vi "MATLAB - Cell Phone Towers.vi"() -> ()   [LabVIEW 2023]
doc: "This example illustrates the use of a Voronoi diagram by using radio towers. After 3 towers are placed, a Voronoi diagram is generated and overlayed to show the area of influence for each tower. It uses the 3D scene graph for display and covers such concepts as object creation, texturing, and transparency. A Voronoi diagram can also be used for path planning and obstacle avoidance in robotics."
panel:
  in  "voronoi output":T1
  out "3D Scene":refnum<vi>(3d-picture)
  in  "Tower height":sgl=3.0
  in  "Maximum amplitude":dbl=0.5
  in  "Size of terrain":i32=50
  in  "Stop":bool
  # "Overview: Illustrates the use of the MATLAB Node to compute a Voronoi diagram with cell phone towers.  After placing three towers, the Voronoi diagram appears.  Each location within a particular region should communicate with the cell phone tower in the same region.\nRequirements: LabVIEW Full Development System, MATLAB(R) Application Software release R2016a or later.\nInstructions:\n1. Run the VI.\n2. Change the view of the image by clicking and dragging. Click <Shift> and drag to zoom. Click <Ctrl> and drag to move the surface. (OS X) Click <Command> and drag to move the surface. \n3. Click <Ctrl-Shift> to create a new cell tower. (OS X) Click <Command-Shift> to create a new cell tower. Add three or more cell towers to see a Voronoi diagram. \n4. Click Stop to stop the VI."
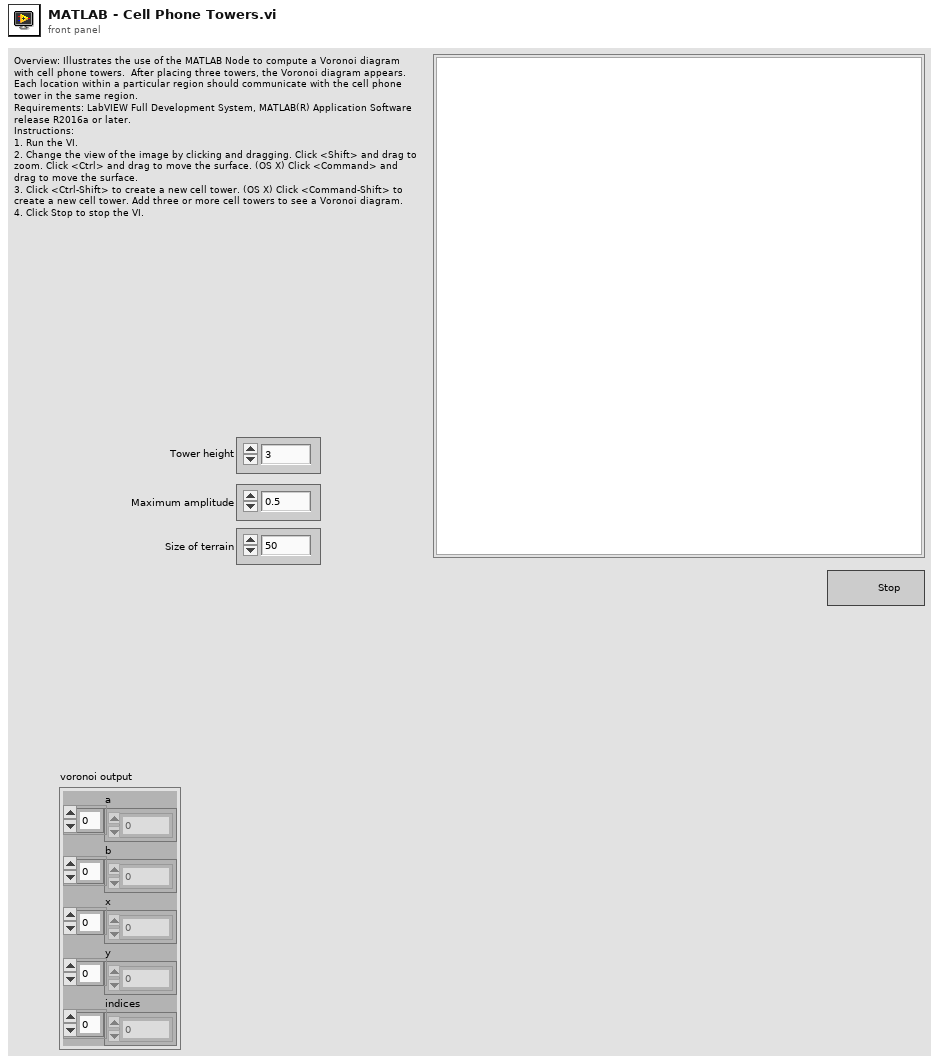
[diagram p1: front panel]
types:
  T1 = cluster{"a":dbl[], "b":dbl[], "x":dbl[], "y":dbl[], "indices":i32[]}
  T2 = typedef "LVPoint32TypeDef.ctl" = cluster{"Horizontal":i32, "Vertical":i32}
  T3 = typedef "LV3DPointTypeDef.ctl" = cluster{"X":sgl, "Y":sgl, "Z":sgl}
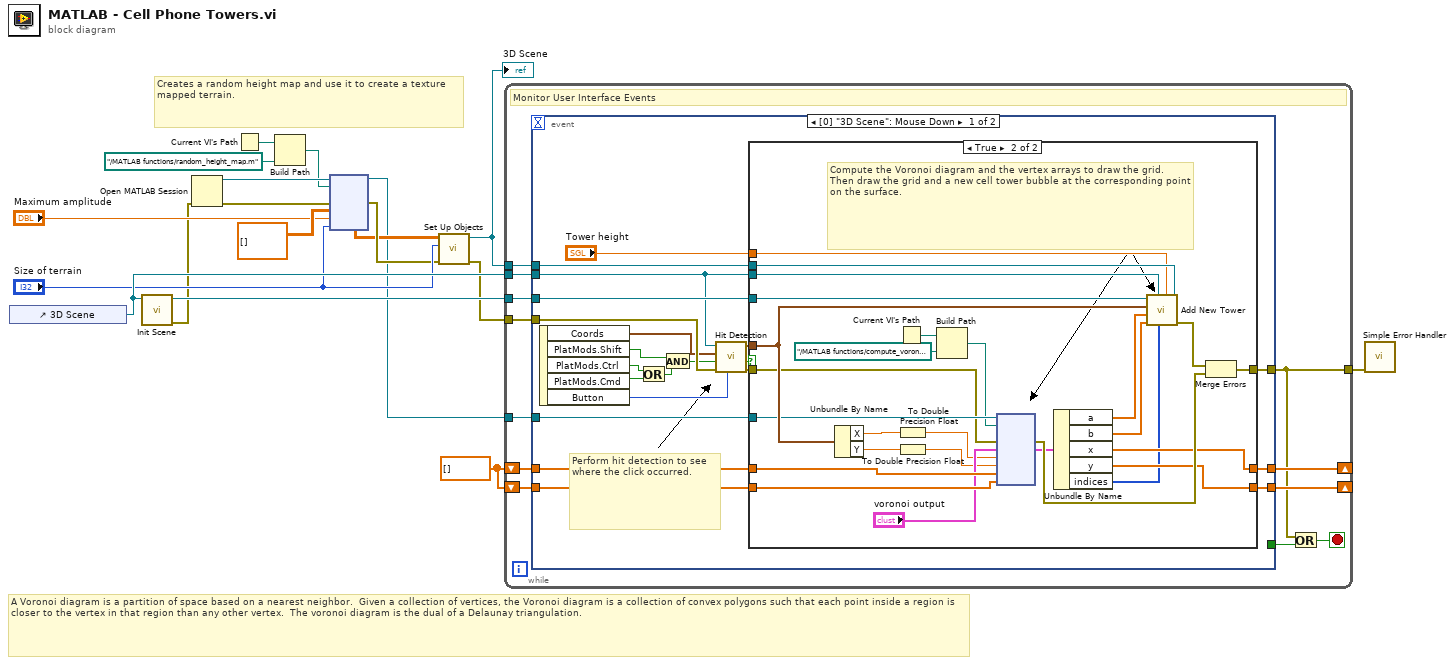
[diagram p0: block diagram]
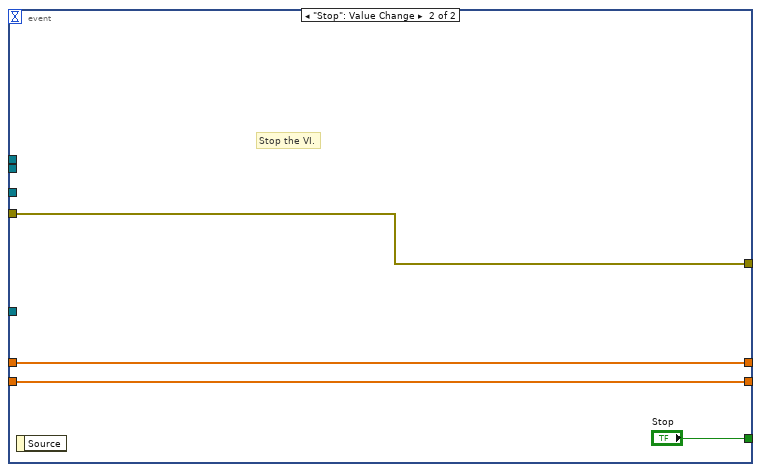
[diagram p3: hidden frame]
diagram:
  w18 = dbl[] []
  # "A Voronoi diagram is a partition of space based on a nearest neighbor.  Given a collection of vertices, the Voronoi diagram is a collection of convex polygons such that each point inside a region is closer to the vertex in that region than any other vertex.  The voronoi diagram is the dual of a Delaunay triangulation."
  # "Creates a random height map and use it to create a texture mapped terrain."
  n1 = control-ref of="3D Scene"() -> (w17:refnum<vi>)
  n2 = call "Init Scene.vi"("SceneGraph Refnum"=w17) -> ("error out"=w4:errorcluster, "Voronoi Grid Object"=w16:refnum<vi>)  [unwired: 9 in]
  n3 = Open MATLAB Session(3:w4) -> (8:w12:refnum<k37>, 11:w11:errorcluster)  [unwired: 1 in]
  n4 = Current VI's Path() -> (path=w10:path)
  n5 = Build Path(base path=w10, name or relative path=path "../MATLAB functions/random_height_map.m") -> (appended path=w8:path)
  n6 = node(w12, w8, w11, dbl[][] [] ("A"), "Maximum amplitude", "Size of terrain") -> (w1:refnum<k37>, w3:errorcluster, w2:dbl[][])  [unwired: 3 in, 2 out]
  n7 = call "Set Up Objects.vi"("error in (no error)"=w3, "len"="Size of terrain", "Height Map"=w2) -> ("error out"=w14:errorcluster, "Main Scene Object Ref (out)"=w15:refnum<vi>)  [unwired: 7 out]
  "3D Scene" <- w15
  n8 = while {
    tunnel: w15 -> [w25]
    shift-right: [w27] -> _
    shift-left: w18 -> [w29]
    shift-right: [w26] -> _
    shift-left: w18 -> [w28]
    tunnel: w17 -> [w24]
    tunnel: w16 -> [w30]
    tunnel: w14 -> [w22]
    tunnel: [w20] -> w13
    tunnel: w1 -> [w19]
    stop <- w21 stop-if-true
    # "Monitor User Interface Events"
    n9 = event shown="[0] \"3D Scene\": Mouse Down" {
      selector: _ -> [_ _]
      dyn-events: _ -> [_ _]
      timeout: _ -> [_ _]
      tunnel: w30 -> [w51 _]
      tunnel: w29 -> [w45 w82]
      tunnel: w28 -> [w44 w81]
      tunnel: [w50 w82] -> w27
      tunnel: [w49 w81] -> w26
      tunnel: w25 -> [w48 _]
      tunnel: w24 -> [w41 _]
      tunnel: [_ "Stop"] -> w23
      tunnel: w22 -> [w39 w83]
      tunnel: [w38 w83] -> w20
      tunnel: w19 -> [w31 _]
      event "3D Scene": Mouse Down {
        # "Perform hit detection to see where the click occurred."
        n10 = event-data() -> ("Coords"=w35:T2, "PlatMods.Shift"=w32:bool, "PlatMods.Ctrl"=w43:bool, "PlatMods.Cmd"=w42:bool, "Button"=w40:u16)  [unwired: 1 out]
        n11 = Or(x=w43, y=w42) -> (x .or. y?=w34:bool)
        n12 = And(x=w32, y=w34) -> (x .and. y?=w33:bool)
        n13 = call "Hit Detection.vi"("Button"=w40, "error in (no error)"=w39, "Alt button?"=w33, "Coords"=w35, "SceneGraphDisp Refnum"=w41) -> ("error out"=w37:errorcluster, "Surface hit?"=w36:bool, "PickPoint"=w46:T3)  [unwired: 4 out]
        n14 = case shown="True" w36 {
          tunnel: w46 -> [_ w79]
          tunnel: "Tower height" -> [_ w77]
          tunnel: w51 -> [_ w80]
          tunnel: w45 -> [w54 w67]
          tunnel: w44 -> [w53 w66]
          tunnel: [w54 w61] -> w50
          tunnel: [w53 w60] -> w49
          tunnel: w48 -> [_ w78]
          tunnel: w41 -> [_ w76]
          tunnel: [w52 w75] -> w38
          tunnel: w37 -> [w52 w69]
          tunnel: w31 -> [_ w71]
          frame False {
          }
          frame True {
            # "Compute the Voronoi diagram and the vertex arrays to draw the grid.  Then draw the grid and a new cell tower bubble at the corresponding point on the surface."
            n15 = Unbundle By Name(w79) -> ("X"=w59:sgl, "Y"=w58:sgl)
            n16 = Current VI's Path() -> (path=w73:path)
            n17 = To Double Precision Float(number=w59) -> (double precision float=w56:dbl)
            n18 = To Double Precision Float(number=w58) -> (double precision float=w57:dbl)
            n19 = Build Path(base path=w73, name or relative path=path "../MATLAB functions/compute_voronoi.m") -> (appended path=w70:path)
            n20 = node(w71, w70, w69, "voronoi output", w56, w57, w67, w66) -> (w68:errorcluster, w64:T1)  [unwired: 5 in, 3 out]
            n21 = Unbundle By Name(w64) -> ("a"=w63:dbl[], "b"=w62:dbl[], "x"=w61:dbl[], "y"=w60:dbl[], "indices"=w55:i32[])
            n22 = call "Add New Tower.vi"("Main Scene Object Ref"=w78, "Tower Height"=w77, "Indices"=w55, "3D Scene reference"=w76, "Voronoi Y vertices"=w62, "Voronoi X vertices"=w63, "Location"=w79, "Voronoi grid ref"=w80) -> ("error out"=w74:errorcluster)  [unwired: 1 in, 2 out]
            n23 = Merge Errors(w74, w68) -> (w75:errorcluster)
          }
        }
      }
      event "Stop": Value Change {
        # "Stop the VI."
        n24 = event-data() -> ()  [unwired: 2 out]
      }
    }
    n25 = Or(x=w20, y=w23) -> (x .or. y?=w21:bool)
  }
  n26 = call <vilib>:"Simple Error Handler.vi"("error in (no error)"=w13) -> ()  [unwired: 4 in, 5 out]
